vi "Initialize Signal.vi"(8 "error in":errorcluster, 10 "Signal":T1 {"Byte Order" items=["Little Endian", "Big Endian"]; "Data Type" items=["Signed", "Unsigned", "IEEE Float"]}, 11 "frame in":refnum<k21>) -> (0 "error out":errorcluster, 2 "signal out":refnum<k21>, 3 "frame out":refnum<k21>)   [LabVIEW 2015, in "Diagnostics Addon Shared.lvlib"]
uses:
  Diagnostics Addon Shared.lvlib
  Types/Signal.ctl
  <vilib>/xnet/xnet.llb/XNET Database Create (Signal).vi
  <resource>/objmgr/xnet.rc
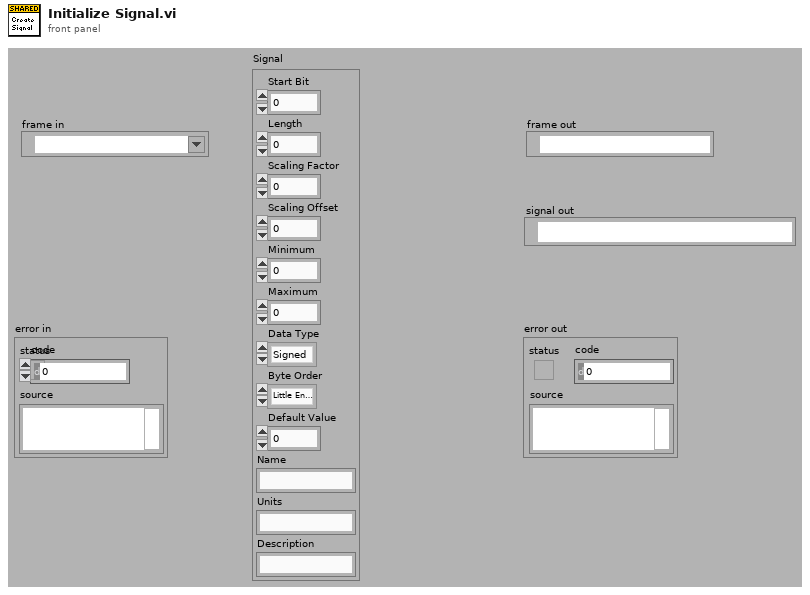
[diagram p1: front panel]
types:
  T1 = typedef "Diagnostics Addon Shared.lvlib/Signal.ctl" = cluster{"Start Bit":u8, "Length":u8, "Scaling Factor":dbl, "Scaling Offset":dbl, "Minimum":dbl, "Maximum":dbl, "Data Type":u32, "Byte Order":u32, "Default Value":dbl, "Name":string, "Units":string, "Description":string}
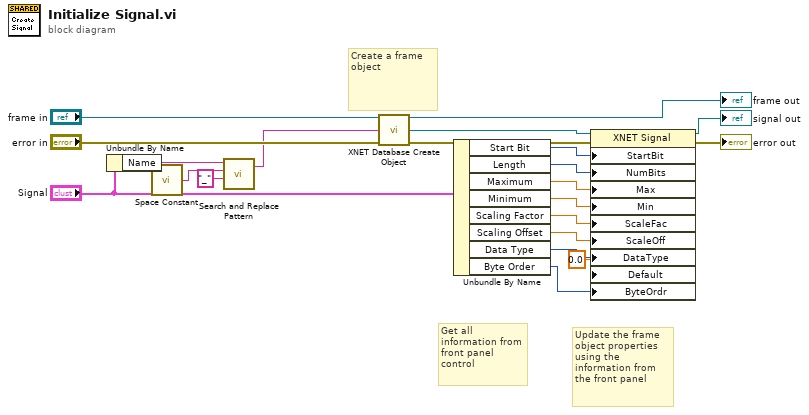
[diagram p0: block diagram]
diagram:
  # "Update the frame object properties using the information from the front panel"
  # "Create a frame object"
  # "Get all information from front panel control"
  n1 = Unbundle By Name("Signal") -> ("Name"=w4:string)
  n2 = call <vilib>:"Space Constant.vi"() -> ("String"=w3:string)
  n3 = call <vilib>:"Search and Replace Pattern.vi"("string"=w4, "regular expression (\"\")"=w3, "replace string (\"\")"="_" ("replace string (\"\")")) -> ("result string"=w5:string)  [unwired: 2 in, 1 out]
  n4 = call-poly <vilib>:"XNET Database Create Object.vi"("frame in"="frame in", "signal name"=w5, "error in (no error)"="error in") -> ("frame out"=→"frame out":refnum<k21>, "signal out"=w17:refnum<k21>, "error out"=w19:errorcluster)  [unwired: 10 in]
  n5 = Unbundle By Name("Signal") -> ("Start Bit"=w15:u8, "Length"=w14:u8, "Maximum"=w13:dbl, "Minimum"=w12:dbl, "Scaling Factor"=w11:dbl, "Scaling Offset"=w10:dbl, "Data Type"=w6:u32, "Byte Order"=w7:u32)
  n6 = property class="XNET Signal"(reference=w17, error in=w19, "StartBit"=w15, "NumBits"=w14, "Max"=w13, "Min"=w12, "ScaleFac"=w11, "ScaleOff"=w10, "DataType"=w6, "Default"=0.0 ("Default Value"), "ByteOrdr"=w7) -> (reference out=→"signal out":refnum<k21>, error out=→"error out":errorcluster)
